vi "String to U32.vi"(8 "error in":errorcluster, 11 "Integer String":string) -> (0 "error out":errorcluster, 3 "U32":u32)   [LabVIEW 2020, in "CANopen.lvlib"]
doc: "Converts the string representation of a number in a specified base to an equivalent 32-bit unsigned integer."
uses:
  CANopen.lvlib
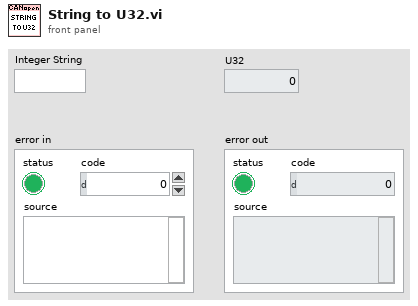
[diagram p1: front panel]
types:
  T1 = enum16{"U8", "U16", "U32", "I8", "I16", "I32", "I64", "U64"}
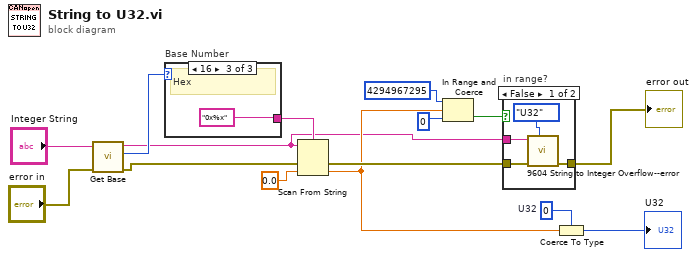
[diagram p0: block diagram]
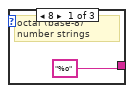
[diagram p3: hidden frame]
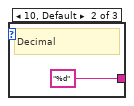
[diagram p4: hidden frame]
diagram:
  w4 = u32 0  # U32
  n1 = call "Get Base.vi"("error in"="error in", "Default Value"="Integer String") -> ("error out"=w11:errorcluster, "Number Base"=w15:u8, "Default Value (dup)"=w1:string)  [unwired: 7 in]
  n2 = case "Base Number" shown="16" w15 {
    tunnel: ["%o" ("format string") "%d" ("format string") "0x%x" ("format string")] -> w13
    frame 8 {
      # "octal (base-8) number strings"
    }
    frame 10, Default {
      # "Decimal"
    }
    frame 16 {
      # "Hex"
    }
  }
  n3 = Scan From String(format string=w13, input string=w1, error in=w11, default 1=0.0 ("DBL")) -> (error out=w8:errorcluster, output 1=w2:dbl)  [unwired: 1 in, 2 out]
  n4 = In Range and Coerce(upper limit=u32 4294967295, x=w2, lower limit=u32 0) -> (In Range?=w6:bool)  [unwired: 1 out]
  n5 = case "in range?" shown="False" w6 {
    tunnel: w8 -> [w22 w23]
    tunnel: [w21 w23] -> w7
    tunnel: w1 -> [w20 _]
    frame False {
      n6 = call "9604 String to Integer Overflow--error.vi"("Type"=T1."U32", "error in"=w22, "Integer String"=w20) -> ("error out"=w21:errorcluster)  [unwired: 8 in]
    }
    frame True {
    }
  }
  "error out" <- w7
  n7 = Coerce To Type(0:w2, 1:w4) -> (2:→"U32":u32)
